vi "UpdateBenchmarkInformation.vi"(8 "error in (no error)":errorcluster, 10 "Benchmark Information in":T1, 11 "VeriStandTestCase in":refnum<class "VeriStandTestCase.lvclass">) -> (0 "error out":errorcluster, 2 "Benchmark Information":T1, 3 "VeriStandTestCase out":refnum<class "VeriStandTestCase.lvclass">)   [LabVIEW 2027, in "VeriStandTestCase.lvclass"]
uses:
  VeriStandTestCase.lvclass
  BenchmarkInformation.ctl
  <vilib>/Analysis/baseanly.llb/Mean (DBL).vi
  <vilib>/Analysis/NI_AALBase.lvlib
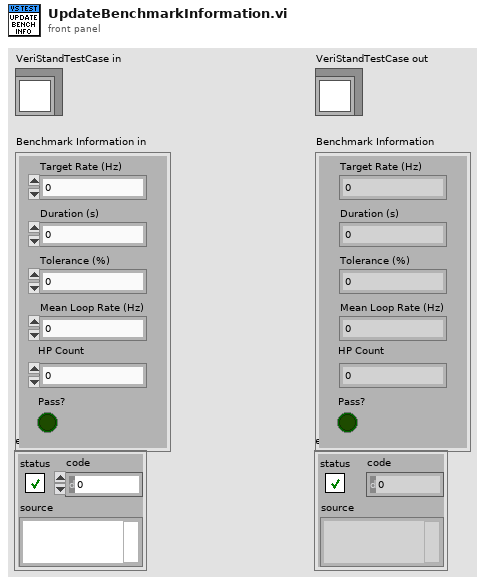
[diagram p1: front panel]
types:
  T1 = typedef "VeriStandTestCase.lvclass/BenchmarkInformation.ctl" = cluster{"Target Rate (Hz)":dbl, "Duration (s)":dbl, "Tolerance (%)":dbl, "Mean Loop Rate (Hz)":dbl, "HP Count":dbl, "Pass?":bool}
  T2 = typedef "VeriStandTestCase.lvclass/SystemChannelInformation.ctl" = cluster{"Actual Loop Rate (Hz)":dbl, "System Time (s)":dbl, "HP Count":dbl, "LP Count":dbl}
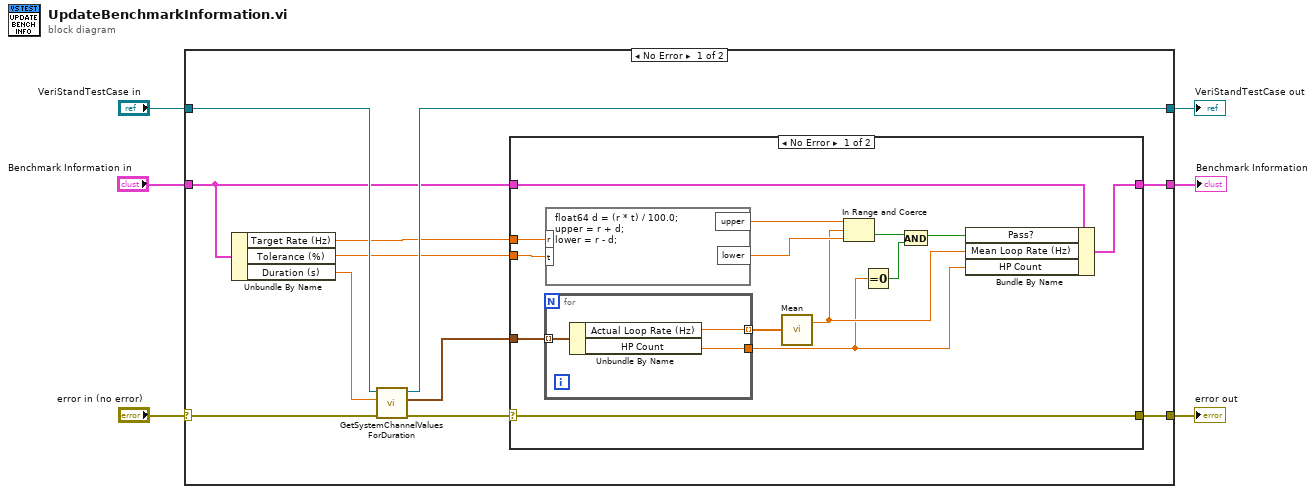
[diagram p0: block diagram]
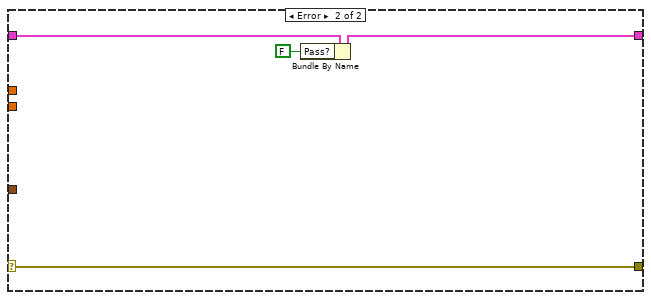
[diagram p2: hidden frame]
diagram:
  n1 = case shown="No Error" "error in (no error)" {
    selector: "error in (no error)" -> [w17 w41]
    tunnel: [w12 w41] -> w5
    tunnel: [w15 w40] -> w3
    tunnel: "VeriStandTestCase in" -> [w16 w40]
    tunnel: [w11 w39] -> w2
    tunnel: "Benchmark Information in" -> [w10 w39]
    frame No Error {
      n2 = Unbundle By Name(w10) -> ("Target Rate (Hz)"=w8:dbl, "Tolerance (%)"=w7:dbl, "Duration (s)"=w14:dbl)
      n3 = call "GetSystemChannelValuesForDuration.vi"("error in (no error)"=w17, "Duration (s)"=w14, "VeriStandTestCase in"=w16) -> ("error out"=w13:errorcluster, "System Channel Information List out"=w9:T2[], "VeriStandTestCase out"=w15:refnum<class "VeriStandTestCase.lvclass">)  [unwired: 6 in]
      n4 = case shown="No Error" w13 {
        selector: w13 -> [w31 w38]
        tunnel: [w31 w38] -> w12
        tunnel: [w20 w36] -> w11
        tunnel: w10 -> [w21 w37]
        tunnel: w9 -> [w30 _]
        tunnel: w8 -> [w28 _]
        tunnel: w7 -> [w27 _]
        frame No Error {
          n5 = for {
            tunnel: w30 -> [w34] mode=indexing
            tunnel: [w33] -> w29 mode=indexing
            tunnel: [w32] -> w18
            n6 = Unbundle By Name(w34) -> ("Actual Loop Rate (Hz)"=w33:dbl, "HP Count"=w32:dbl)
          }
          n7 = formula code="float64 d = (r * t) / 100.0;\nupper = r + d;\nlower = r - d;"("r"=w28, "t"=w27) -> ("upper"=w26:dbl, "lower"=w25:dbl)
          n8 = call-poly <vilib>:"Mean.vi"("X"=w29) -> ("mean"=w24:dbl)  [unwired: 1 out]
          n9 = In Range and Coerce(upper limit=w26, x=w24, lower limit=w25) -> (In Range?=w23:bool)  [unwired: 1 out]
          n10 = Equal To 0?(x=w18) -> (x = 0?=w19:bool)
          n11 = And(x=w23, y=w19) -> (x .and. y?=w22:bool)
          n12 = Bundle By Name(cluster=w21, "Pass?"=w22, "Mean Loop Rate (Hz)"=w24, "HP Count"=w18) -> (w20:T1)
        }
        frame Error {
          n13 = Bundle By Name(cluster=w37, "Pass?"=FALSE) -> (w36:T1)
        }
      }
    }
    frame Error {
    }
  }
  "error out" <- w5
  "VeriStandTestCase out" <- w3
  "Benchmark Information" <- w2
